vi "Elapsed_time.vi"() -> ()   [LabVIEW 2020]
panel:
  out "millisecond timer value":u32
  in  "milliseconds to wait":u32
  out "Time has Elapsed":bool
  in  "Auto Reset":bool=TRUE
  in  "Reset":bool
  in  "Time Target (s)":dbl=1.0
  out "Elapsed Time (s)":dbl
  out "# Ramdom":dbl
  out "Numero de iteraciones":dbl
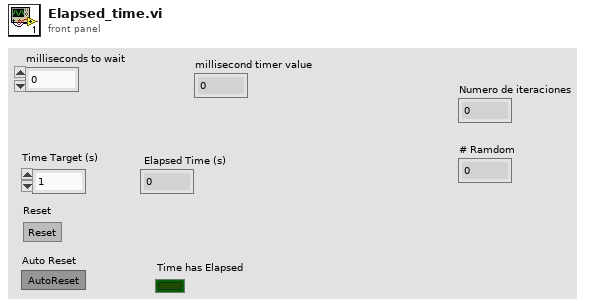
[diagram p1: front panel]
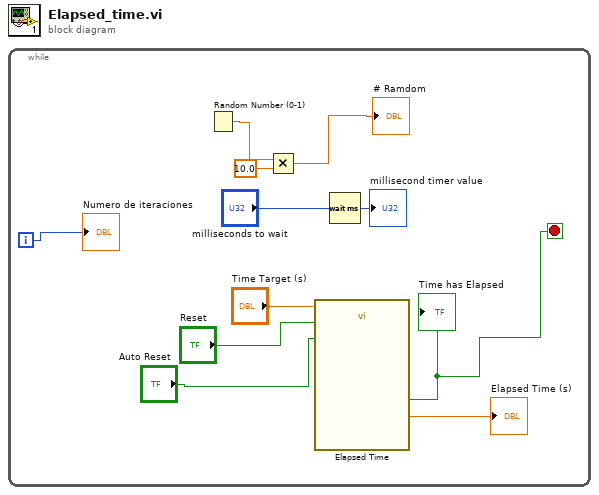
[diagram p0: block diagram]
diagram:
  n1 = while {
    i -> [w9]
    stop <- w3 stop-if-true
    n2 = Random Number (0-1)() -> (number: 0 to 1=w11:dbl)
    n3 = Multiply(x=w11, y=10.0) -> (x*y=→"# Ramdom":dbl)
    n4 = call "Elapsed Time"("Time Target (s)"="Time Target (s)", "Reset"="Reset", "Auto Reset"="Auto Reset") -> ("Elapsed Time (s)"=→"Elapsed Time (s)":dbl, "Time has Elapsed"=w3:bool)  [unwired: 9 in, 6 out]
    "Time has Elapsed" <- w3
    n5 = Wait (ms)(milliseconds to wait="milliseconds to wait") -> (millisecond timer value=→"millisecond timer value":u32)
    "Numero de iteraciones" <- w9
  }
